vi "Arduino Leonardo.vi"() -> (0 "Arduino Leonardo":T1={"DI Channels"=[2, 3, 4, 5, 6, 7, 8, 9, 10, 11, 12, 13], "DO Channels"=[2, 3, 4, 5, 6, 7, 8, 9, 10, 11, 12, 13], "AI"=[0, 1, 2, 3, 4, 5], "AO"=[], "PWM"=[3, 5, 6, 9, 10, 11], "QE"=[], "UART"=[], "I2C 2"=[0], "SPI"=[0], "CAN"=[], "AI Ref (V)"=5.0, "Firmware Program Interfaces"=[enum."Serial / USB"], "Firmware Versions"=[{"Name"="LINX -  Serial / USB ", "Relative Path"="\\Arduino\\Leonardo\\Leonardo_Serial_USB.hex", "Firmware Interface"=enum."Serial "}], "Name"="Arduino Leonardo", "AO Resolution (Bits)"=0, "AO Ref (V)"=0.0})   [LabVIEW 2014, in "LMH-LINX.lvlib"]
uses:
  <vilib>/MakerHub/LINX/LMH-LINX.lvlib
  <vilib>/MakerHub/LINX/Private/Type Defs/Devices/Generic Device.ctl
  <vilib>/MakerHub/LINX/Private/Type Defs/Firmware Version.ctl
  <vilib>/MakerHub/LINX/Private/Device/Type Defs/Firmware Interface.ctl
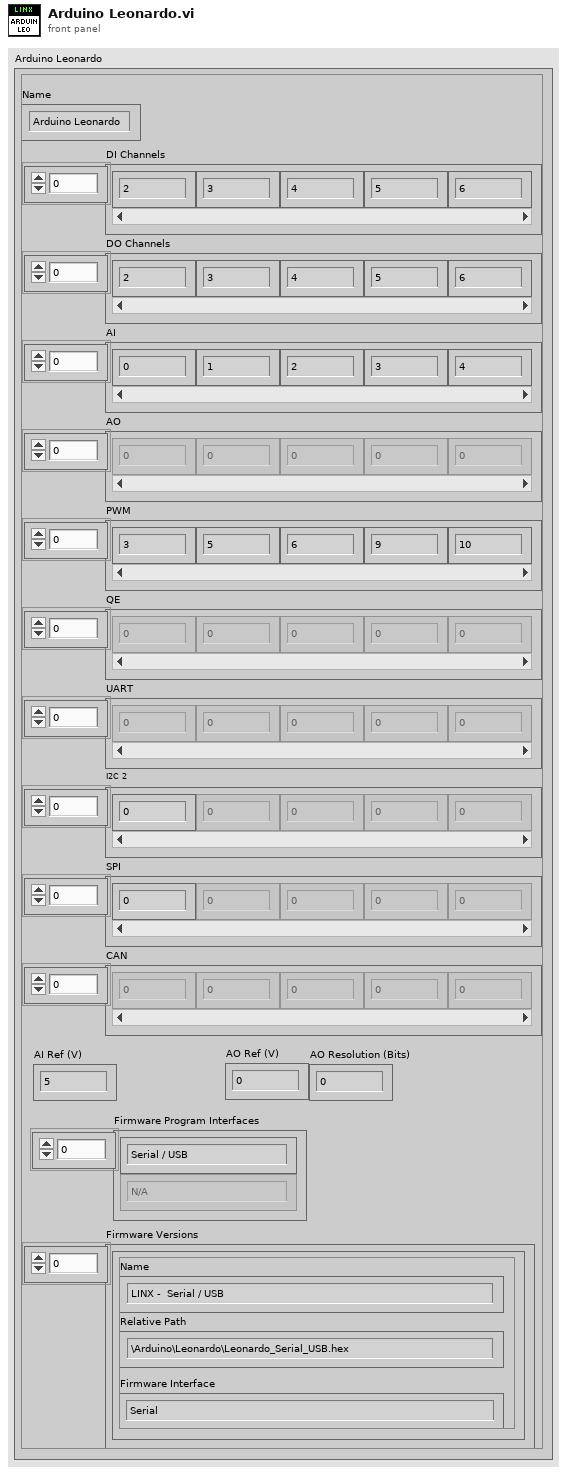
[diagram p1: front panel]
types:
  T1 = typedef "LMH-LINX.lvlib/Generic Device.ctl" = cluster{"DI Channels":u8[], "DO Channels":u8[], "AI":u8[], "AO":u8[], "PWM":u8[], "QE":u8[], "UART":u8[], "I2C 2":u8[], "SPI":u8[], "CAN":u8[], "AI Ref (V)":dbl, "Firmware Program Interfaces":enum16{"N/A", "Serial / USB", "USB", "TCP"}[], "Firmware Versions":T2[], "Name":string, "AO Resolution (Bits)":u8, "AO Ref (V)":dbl}
  T2 = typedef "LMH-LINX.lvlib/Firmware Version.ctl" = cluster{"Name":string, "Relative Path":string, "Firmware Interface":T3}
  T3 = typedef "LMH-LINX.lvlib/Firmware Interface.ctl" = enum32{"Serial ", "Ethernet", "WIFI"}
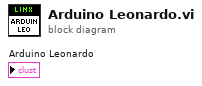
[diagram p0: block diagram]
diagram:
